vi "That was easy new VI test.vi"() -> ()   [LabVIEW 2009]
uses:
  <vilib>/userDefined/High Color/nirio_resource_hc.ctl
  <vilib>/rvi/interface/nirviOpenFPGA/nirviOpenFPGA.xnode
  FPGA Bitfiles/Q_IGVC_2010.lvproj_FPGA Target_FPGA_MAIN.vi.lvbitx
  <vilib>/FPGAPlugInAG/cRIO-9113/nirviIntfOpen_cRIO-9113.vi
  <vilib>/rvi/interface/nirviCloseFPGA/nirviCloseFPGA.xnode
  <vilib>/FPGAPlugInAG/cRIO-9113/nirviIntfClose_cRIO-9113.vi
  TypeDefs/Sensor Typedefs/FPGA Main ref.ctl
panel:
  out "error out":errorcluster
  in  "stop":bool
  in  "That was easy!":bool
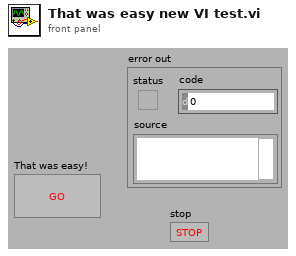
[diagram p1: front panel]
types:
  T1 = typedef "nirio_resource_hc.ctl" = tag
  T2 = typedef "FPGA Main ref.ctl" = refnum<k20>
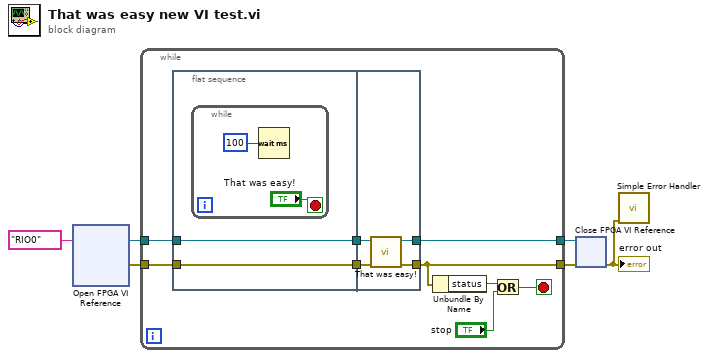
[diagram p0: block diagram]
diagram:
  n1 = xnode "Open FPGA VI Reference"("resource name"=T1 "RIO0") -> ("FPGA VI Reference Out"=w6:T2, "error out"=w5:errorcluster)  [unwired: 1 in]
  n2 = while {
    tunnel: w6 -> [w13]
    tunnel: w5 -> [w12]
    tunnel: [w11] -> w4
    tunnel: [w8] -> w3
    stop <- w9 stop-if-true
    n3 = flat-sequence {
      tunnel: w12 -> [w16]
      tunnel: w13 -> [w17]
      tunnel: [w17] -> w15
      tunnel: [w16] -> w14
      tunnel: w15 -> [w23]
      tunnel: w14 -> [w22]
      tunnel: [w21] -> w11
      tunnel: [w20] -> w8
      frame #0 {
        n4 = while {
          stop <- "That was easy!" stop-if-true
          n5 = Wait (ms)(milliseconds to wait=u32 100) -> ()  [unwired: 1 out]
        }
      }
      frame #1 {
        n6 = call "That was easy!.vi"("error in (no error)"=w22, "FPGA VI Reference in"=w23) -> ("error out"=w20:errorcluster, "FPGA VI Reference out"=w21:T2)  [unwired: 8 in]
      }
    }
    n7 = Unbundle By Name(w8) -> ("status"=w7:bool)
    n8 = Or(x=w7, y="stop") -> (x .or. y?=w9:bool)
  }
  n9 = xnode "Close FPGA VI Reference"("FPGA VI Reference In"=w4, "error in"=w3) -> ("error out"=w1:errorcluster)
  "error out" <- w1
  n10 = call <vilib>:"Simple Error Handler.vi"("error in (no error)"=w1) -> ()  [unwired: 4 in, 5 out]
